vi "Get Node List.vi"(8 "error in (no error)":errorcluster, 11 "INI Deserializer in":refnum<class "INI Deserializer.lvclass">) -> (0 "error out":errorcluster, 1 "Subnodes":string[](array[string]), 2 "Root Node":string)   [LabVIEW 2014, in "INI Deserializer.lvclass"]
uses:
  INI Deserializer.lvclass
  INI Deserializer.lvclass/INI Deserializer.ctl
  <vilib>/Utility/config.llb/NI_LVConfig.lvlib
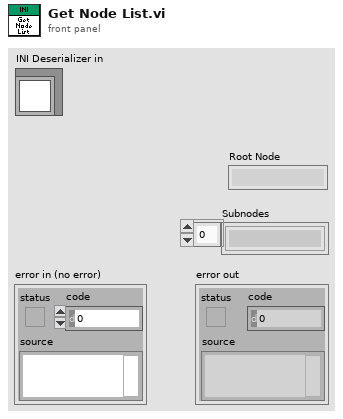
[diagram p1: front panel]
types:
  T1 = typedef "NI_LVConfig.lvlib/Config Data RefNum.ctl" = refnum<k1>
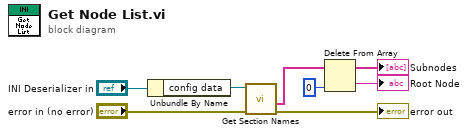
[diagram p0: block diagram]
diagram:
  n1 = Unbundle By Name("INI Deserializer in") -> ("config data"=w6:T1)
  n2 = call <vilib>:"Get Section Names.vi"("error in (no error)"="error in (no error)", "refnum"=w6) -> ("error out"=→"error out":errorcluster, "section names"=w2:string[])  [unwired: 7 in, 1 out]
  n3 = Delete From Array(array=w2, index=0) -> (deleted portion=→"Root Node":string, array with subset deleted=→"Subnodes":string[])  [unwired: 1 in]
